vi "Controle_Motor.vi"(0 "stop":bool, 1 "Enable":bool, 2 "Direção  2":bool, 3 "Enable 2":tag, 4 "Timer Reset":bool, 5 "Direção":tag, 7 "Pulso":tag, 9 "Constante Calibracao (mm/pulsos)":dbl, 10 "Velocidade ( mm/s )":dbl, 11 "Distancia (mm)":dbl) -> ()   [LabVIEW 2025]
uses:
  <vilib>/DAQmx/create/channels.llb/DAQmx Create Channel (DO-Digital Output).vi
  <vilib>/DAQmx/create/channels.llb/DAQmx Create Channel (CO-Pulse Generation-Frequency).vi
  <vilib>/DAQmx/configure/timing.llb/DAQmx Timing (Implicit).vi
  <vilib>/DAQmx/write.llb/DAQmx Write (Digital Bool 1Line 1Point).vi
panel:
  in  "Tab Control":enum32{"Atuador", "Configuração das Portas"}(tab)
  out "Loop Count":i32
  out "Elapsed Time (s)":dbl
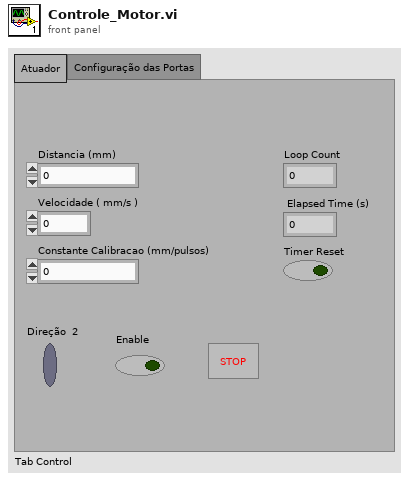
[diagram p1: front panel]
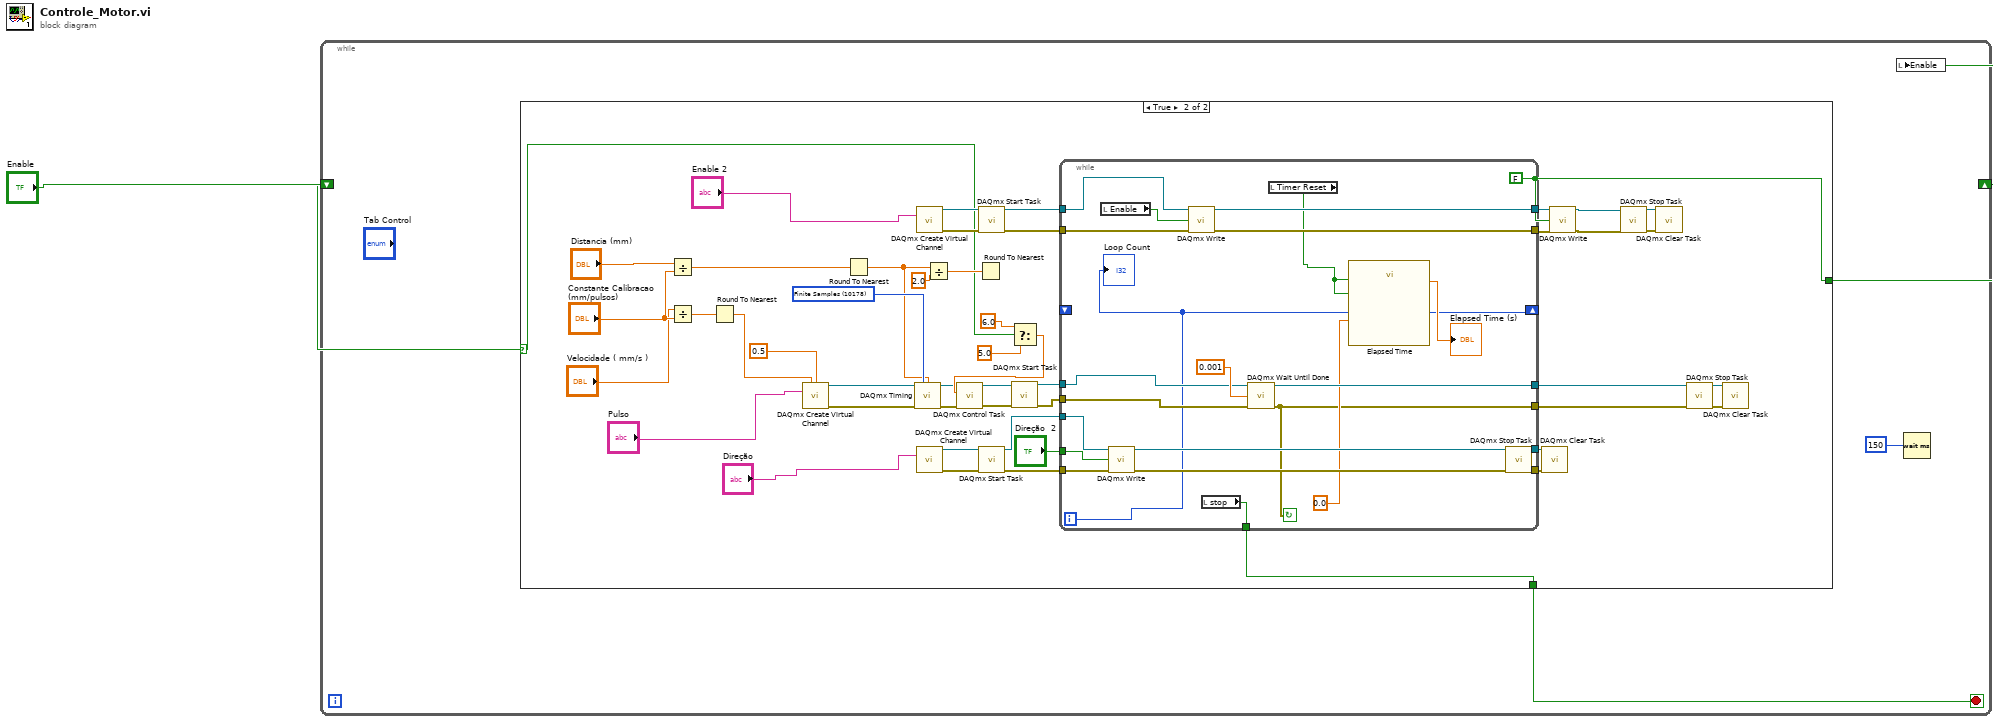
[diagram p0: block diagram]
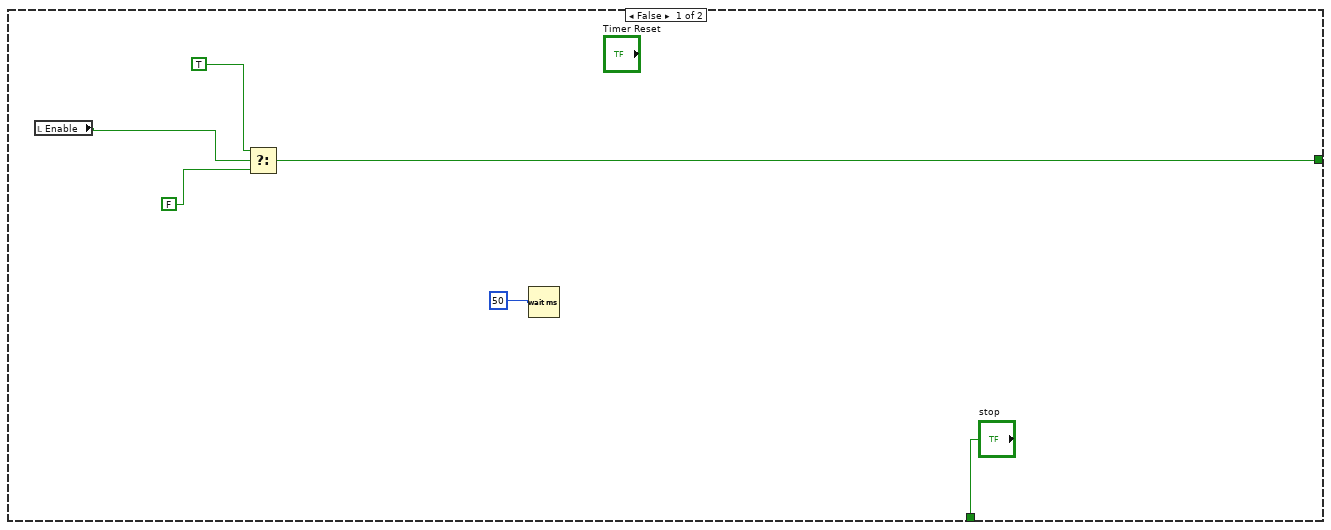
[diagram p2: hidden frame]
diagram:
  n1 = while {
    shift-right: [w4] -> _
    shift-left: "Enable" -> [w5]
    stop <- w2 stop-if-true
    n2 = case shown="True" w5 {
      selector: w5 -> [_ w18]
      tunnel: [w7 w13] -> w4
      tunnel: ["stop" w12] -> w2
      frame False {
        n3 = local read "Enable"() -> (w8:bool)
        n4 = Select(t=TRUE, s=w8, f=FALSE) -> (s? t:f=w7:bool)
        n5 = Wait (ms)(milliseconds to wait=u32 50) -> ()  [unwired: 1 out]
      }
      frame True {
        w13 = FALSE ("data")
        w46 = 10178 items=["Finite Samples"=10178, "Continuous Samples"=10123, "Hardware Timed Single Point"=12522] ("sample mode")
        n6 = Divide(x="Distancia (mm)", y="Constante Calibracao (mm/pulsos)") -> (x/y=w38:dbl)
        n7 = Divide(x="Velocidade ( mm/s )", y="Constante Calibracao (mm/pulsos)") -> (x/y=w36:dbl)
        n8 = Round To Nearest(number=w36) -> (nearest integer value=w34:dbl)
        n9 = call-poly <vilib>:"DAQmx Create Virtual Channel.vi"("frequency"=w34, "duty cycle"=0.5, "counter"="Pulso") -> ("task out"=w48:refnum<k21>, "error out"=w47:errorcluster)  [unwired: 11 in]
        n10 = Round To Nearest(number=w38) -> (nearest integer value=w37:dbl)
        n11 = call-poly <vilib>:"DAQmx Timing.vi"("task/channels in"=w48, "sample mode"=w46, "samples per channel"=w37, "error in"=w47) -> ("task out"=w24:refnum<k21>, "error out"=w19:errorcluster)  [unwired: 10 in]
        n12 = call-poly <vilib>:"DAQmx Create Virtual Channel.vi"("lines"="Enable 2") -> ("task out"=w60:refnum<k21>, "error out"=w61:errorcluster)  [unwired: 13 in]
        n13 = call-poly <vilib>:"DAQmx Create Virtual Channel.vi"("lines"="Direção") -> ("task out"=w62:refnum<k21>, "error out"=w59:errorcluster)  [unwired: 13 in]
        n14 = Divide(x=w37, y=2.0) -> (x/y=w35:dbl)
        n15 = Round To Nearest(number=w35) -> ()  [unwired: 1 out]
        n16 = call <vilib>:"DAQmx Start Task.vi"("task/channels in"=w60, "error in"=w61) -> ("task out"=w56:refnum<k21>, "error out"=w55:errorcluster)  [unwired: 12 in]
        n17 = call <vilib>:"DAQmx Start Task.vi"("task/channels in"=w62, "error in"=w59) -> ("task out"=w58:refnum<k21>, "error out"=w57:errorcluster)  [unwired: 12 in]
        n18 = Select(t=6.0 ("y"), s=w18, f=5.0 ("y")) -> (s? t:f=w25:dbl)
        n19 = call <vilib>:"DAQmx Control Task.vi"("task/channels in"=w24, "action"=w25, "error in"=w19) -> ("task out"=w23:refnum<k21>, "error out"=w20:errorcluster)  [unwired: 11 in]
        n20 = call <vilib>:"DAQmx Start Task.vi"("task/channels in"=w23, "error in"=w20) -> ("task out"=w22:refnum<k21>, "error out"=w21:errorcluster)  [unwired: 12 in]
        n21 = while {
          tunnel: w58 -> [w82]
          tunnel: w57 -> [w81]
          tunnel: w56 -> [w80]
          tunnel: w55 -> [w79]
          tunnel: [w78] -> w50
          tunnel: [w77] -> w49
          tunnel: [w76] -> w16
          tunnel: [w75] -> w14
          tunnel: "Direção  2" -> [w74]
          tunnel: [w70] -> w32
          tunnel: [w67] -> w31
          shift-right: [w66] -> _
          shift-left: _ -> [_]
          tunnel: w21 -> [w72]
          tunnel: w22 -> [w71]
          tunnel: [w65] -> w12
          i -> [w66]
          stop <- w67 continue-if-true
          n22 = local read "Enable"() -> (w63:bool)
          n23 = call-poly <vilib>:"DAQmx Write.vi"("task/channels in"=w82, "data"=w74, "error in"=w81) -> ("task out"=w78:refnum<k21>, "error out"=w77:errorcluster)  [unwired: 10 in, 1 out]
          n24 = call-poly <vilib>:"DAQmx Write.vi"("task/channels in"=w80, "data"=w63, "error in"=w79) -> ("task out"=w76:refnum<k21>, "error out"=w75:errorcluster)  [unwired: 10 in, 1 out]
          n25 = local read "stop"() -> (w65:bool)
          n26 = call <vilib>:"DAQmx Wait Until Done.vi"("task/channels in"=w71, "timeout (sec)"=0.001 ("y"), "error in"=w72) -> ("task out"=w70:refnum<k21>, "error out"=w67:errorcluster)  [unwired: 11 in]
          n27 = local read "Timer Reset"() -> (w64:bool)
          n28 = call "Elapsed Time"("Reset"=w64, "Auto Reset"=w64, "Set Start Time (s)"=0.0) -> ("Elapsed Time (s)"=→"Elapsed Time (s)":dbl)  [unwired: 9 in, 7 out]
          "Loop Count" <- w66
        }
        n29 = call <vilib>:"DAQmx Stop Task.vi"("task/channels in"=w50, "error in"=w49) -> ("task out"=w54:refnum<k21>, "error out"=w53:errorcluster)  [unwired: 12 in]
        n30 = call <vilib>:"DAQmx Clear Task.vi"("task in"=w54, "error in"=w53) -> ()  [unwired: 13 in, 1 out]
        n31 = call-poly <vilib>:"DAQmx Write.vi"("task/channels in"=w16, "data"=w13, "error in"=w14) -> ("task out"=w17:refnum<k21>, "error out"=w15:errorcluster)  [unwired: 10 in, 1 out]
        n32 = call <vilib>:"DAQmx Stop Task.vi"("task/channels in"=w17, "error in"=w15) -> ("task out"=w52:refnum<k21>, "error out"=w51:errorcluster)  [unwired: 12 in]
        n33 = call <vilib>:"DAQmx Clear Task.vi"("task in"=w52, "error in"=w51) -> ()  [unwired: 13 in, 1 out]
        n34 = call <vilib>:"DAQmx Stop Task.vi"("task/channels in"=w32, "error in"=w31) -> ("task out"=w44:refnum<k21>, "error out"=w43:errorcluster)  [unwired: 12 in]
        n35 = call <vilib>:"DAQmx Clear Task.vi"("task in"=w44, "error in"=w43) -> ()  [unwired: 13 in, 1 out]
      }
    }
    n36 = local write "Enable"(w4) -> ()
    n37 = Wait (ms)(milliseconds to wait=u32 150) -> ()  [unwired: 1 out]
  }
